vi "TL midbrain SENSE.vi"(5 "Last location":cluster{"X pos":i32, "Y pos":i32, "Heading":dbl}, 6 "Boat Status":T2, 7 "error in":errorcluster) -> (0 "Last location out":cluster{"X pos":i32, "Y pos":i32, "Heading":dbl}, 1 "Stuck?":bool, 2 "Battery\nDead?":bool, 3 "error out":errorcluster, 4 "IR Sensors":T1)   [LabVIEW 2014]
doc: "This VI receives the status of the boat from the Hindbrain and determines:\n1. Is the boat stuck?\n2. Is the battery dead?"
uses:
  boatStatus.ctl
  sensorsSTD.ctl
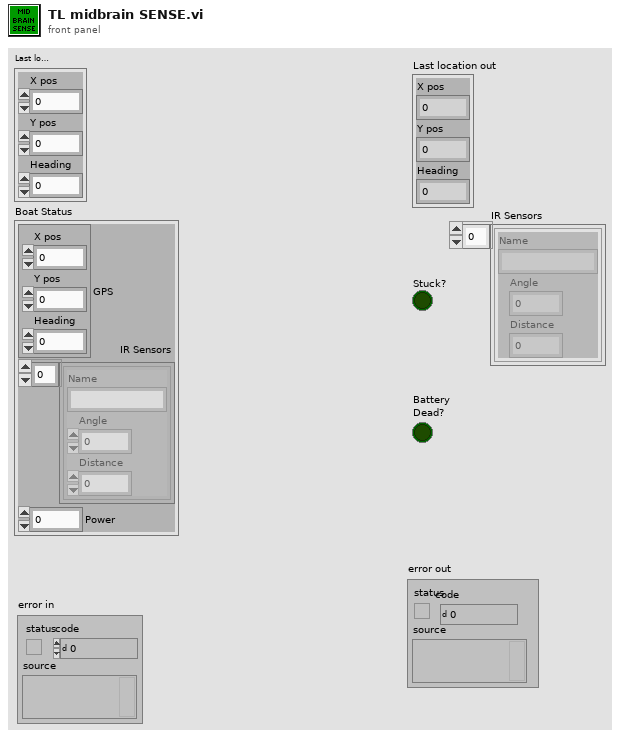
[diagram p1: front panel]
types:
  T1 = typedef "sensorsSTD.ctl" = cluster{"Name":string, "Angle":dbl, "Distance":dbl}[]
  T2 = typedef "boatStatus.ctl" = cluster{"GPS":cluster{"X pos":i32, "Y pos":i32, "Heading":dbl}, "IR Sensors":cluster{"Name":string, "Angle":dbl, "Distance":dbl}[], "Power":dbl}
  T3 = cluster{"Name":string, "Angle":dbl, "Distance":dbl}[]
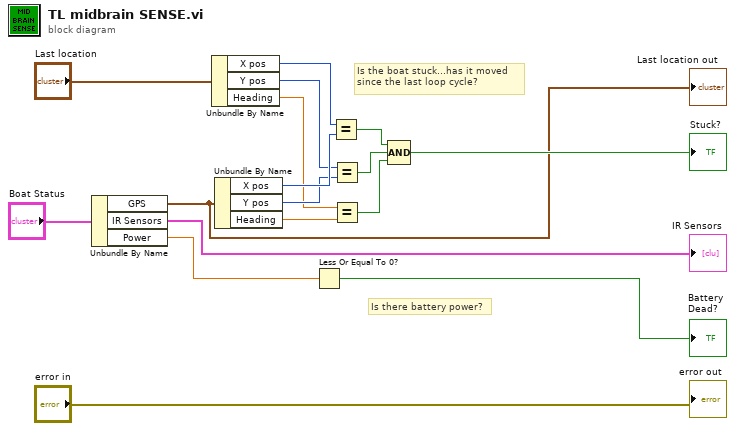
[diagram p0: block diagram]
diagram:
  # "Is there battery power?"
  # "Is the boat stuck...has it moved \nsince the last loop cycle?"
  n1 = Unbundle By Name("Boat Status") -> ("GPS"=w9:cluster{"X pos":i32, "Y pos":i32, "Heading":dbl}, "IR Sensors"=→"IR Sensors":T3, "Power"=w8:dbl)
  "Last location out" <- w9
  n2 = Unbundle By Name("Last location") -> ("X pos"=w15:i32, "Y pos"=w13:i32, "Heading"=w3:dbl)
  n3 = Unbundle By Name(w9) -> ("X pos"=w14:i32, "Y pos"=w12:i32, "Heading"=w4:dbl)
  n4 = Less Or Equal To 0?(x=w8) -> (x <= 0?=→"Battery\nDead?":bool)
  n5 = Equal?(x=w15, y=w14) -> (x = y?=w11:bool)
  n6 = Equal?(x=w13, y=w12) -> (x = y?=w6:bool)
  n7 = Equal?(x=w3, y=w4) -> (x = y?=w5:bool)
  n8 = Compound Arithmetic op=AND(w11, w6, w5) -> (→"Stuck?":bool)
  "error out" <- "error in"
